vi "IIR Filter with I.C. (CDB).vi"(5 "Initial Y Conditions":cdb[](array[numeric]), 6 "Initial X Conditions":cdb[](array[numeric]), 7 "Forward Coefficients":dbl[](array[numeric]), 9 "Reverse Coefficients":dbl[](array[numeric]), 10 "X":cdb[](array[numeric])) -> (0 "Final X Conditions":cdb[](array[numeric]), 1 "Final Y Conditions":cdb[](array[numeric]), 2 "error":i32, 3 "Filtered X":cdb[](array[numeric]))   [LabVIEW 2018, in "NI_AALBase.lvlib"]
doc: "Filters the input sequence <B>X</B> using the direct form IIR filter specified by <B>Reverse Coefficients</B> and <B>Forward Coefficients</B>. You can use this VI to process blocks of continuous data. This VI is similar to the IIR Filter VI except that you specify the initial conditions for this VI. Wire data to the <B>X</B> input to determine the polymorphic instance to use or manually select the instance."
uses:
  <vilib>/Analysis/NI_AALBase.lvlib
  <resource>/lvanlys.dll
panel:
  # "IIR Filter with I.C."
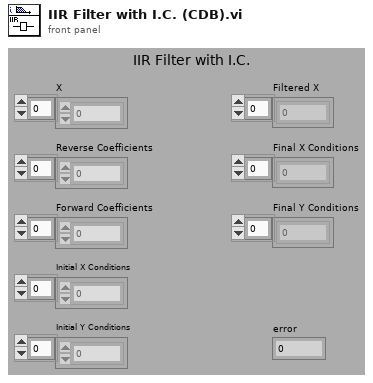
[diagram p1: front panel]
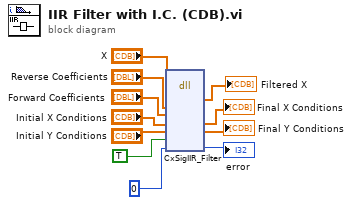
[diagram p0: block diagram]
diagram:
  n1 = dll-call lib="C:/Program Files (x86)/National Instruments/LabVIEW 2018/resource/lvanlys.*" fn="CxSigIIR_Filter"("X"="X", "aH"="Reverse Coefficients", "bH"="Forward Coefficients", "Initial X Conditions"="Initial X Conditions", "Initial Y Conditions"="Initial Y Conditions", TRUE, "dsperr"=0) -> ("X"=→"Filtered X":cdb[], "Initial X Conditions"=→"Final X Conditions":cdb[], "Initial Y Conditions"=→"Final Y Conditions":cdb[], "dsperr"=→"error":i32)  [unwired: 7 in, 2 out]
